vi "Untitled 2.vi"() -> ()   [LabVIEW 2020]
uses:
  HAL/Source/Communicator/Communicator.lvclass
  D:/git/HAL/Source/Interfaces/ICommunicate/ICommunicate.lvclass
  HAL/HAL-Devices/source/PCAN USB Dongle/PCAN Basic 4/Configure Strategies/Read-Write CAN Frame Strategy/PCAN Basic4 Read-Write CAN CC Frame Strategy.lvclass
  D:/git/HAL/Source/Interfaces/IConfigure/IConfigure.lvclass
  HAL/Source/Interfaces/IMessage/IMessage.lvclass
  source/SDO Manager/SDO Manager/SDO Manager.lvclass
  source/SDO Manager/SDO Transfer/SDO abort code.ctl
  source/SDO Manager/SDO Transfer/SDO Transfer.lvclass
  source/Typedefs/SDO Result.ctl
  source/CANopen.lvlib
panel:
  out "(hi.lo)":u32
  out "Data R":u8[](array[numeric]) format="%x"
  out "Data S":u8[](array[numeric]) format="%x"
  out "SDO Result":T1={"Success"=FALSE, "SDO abort code"={"Null"=TRUE, "Value"=84082688}, "Data"={"Null"=TRUE, "Data"=[]}} {"SDO abort code"."Value" items=["Toggle bit not allowed"=84082688, "SDO protocol timed out"=84148224, "Client/server command specifier not valid or unknown"=84148225, "Invalid block size (block mode only)"=84148226, "Invalid sequence number (block mode only)"=84148227, "CRC error (block mode only)"=84148228, "Out of memory"=84148229, "Attempt to read a write only object"=100728833, "Attempt to write a read only object"=100728834, "Object does not exist in the object dictionary"=100794368, "Object cannot be mapped to the PDO"=100925505, "The number and length of the objects to be mapped would exceed PDO length"=100925506, "General parameter incompatibility reason"=100925507, "General internal incompatibility in the device"=100925511, "Access failed due to an hardware error"=101056512, "Data type does not match, length of service parameter does not match"=101122064, "Data type does not match, length of service parameter too high"=101122066, "Data type does not match, length of service parameter too low"=101122067, "Sub-index does not exist"=101253137, "Invalid value for parameter (download only)"=101253168, "Value of parameter written too high (download only)"=101253169, "Value of parameter written too low (download only)"=101253170, "Maximum value is less than minimum value"=101253174, "Resource not available: SDO connection"=101318691, "General error"=134217728, "Data cannot be transferred or stored to the application"=134217760, "Data cannot be transferred or stored to the application because of local control"=134217761, "Data cannot be transferred or stored to the application because of the present device stable"=134217762, "Object dictionary dynamic generation fails or no object dictionary is present (e.g. object dictionary is generated from file and generation fails because of an file error)"=134217763, "No data available"=134217764]; "Data"."Data" format="%02x"}
  out "error out":errorcluster
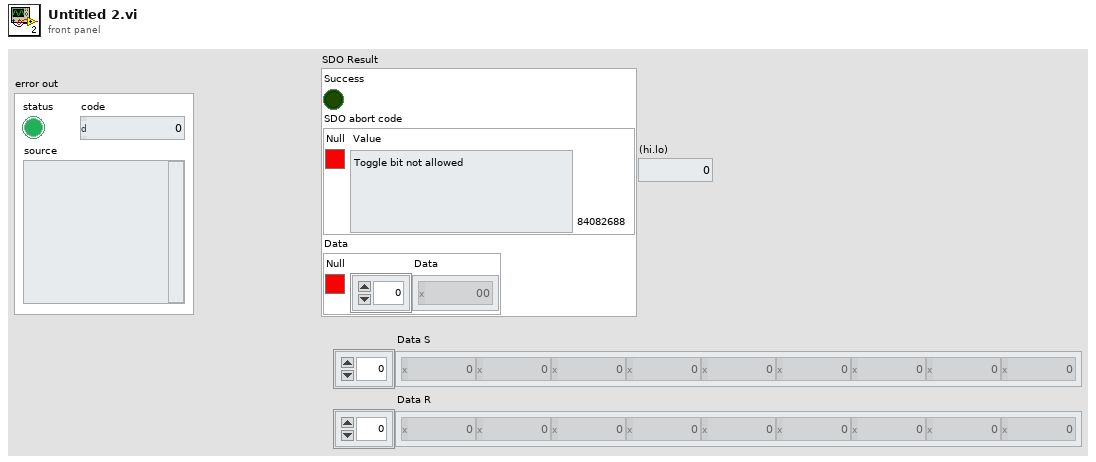
[diagram p1: front panel]
types:
  T1 = typedef "CANopen.lvlib/SDO Result.ctl" = cluster{"Success":bool, "SDO abort code":cluster{"Null":bool, "Value":T2}, "Data":cluster{"Null":bool, "Data":u8[]}}
  T2 = typedef "SDO Manager.lvlib/SDO Transfer.lvclass/SDO abort code.ctl" = u32
  T3 = cluster{"Node-ID":u8, "Multiplexer":cluster{"Index":u16, "Sub-Index":u8}, "Data":u8[]}
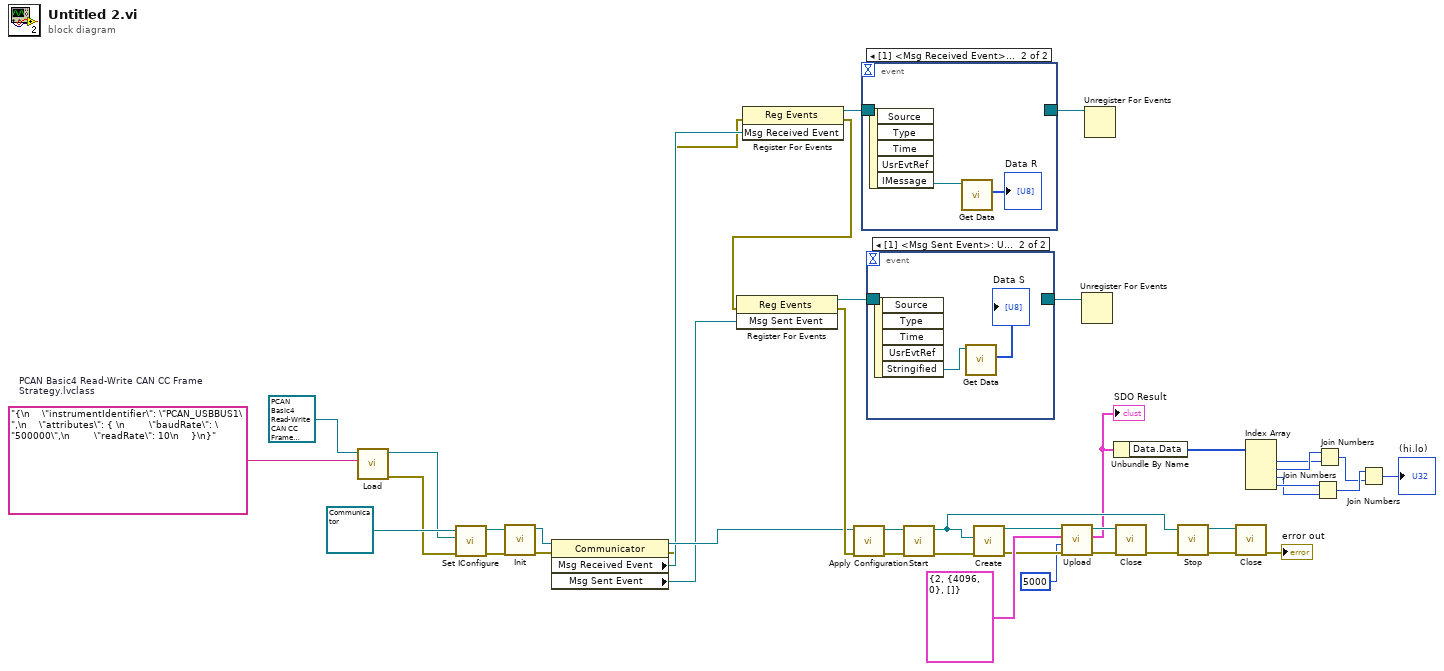
[diagram p0: block diagram]
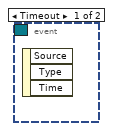
[diagram p2: hidden frame]
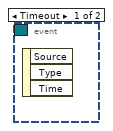
[diagram p3: hidden frame]
diagram:
  w42 = refnum<class "PCAN Basic4 Read-Write CAN CC Frame Strategy.lvclass"> refnum  # PCAN Basic4 Read-Write CAN CC Frame Strategy.lvclass
  n1 = call-dynamic "Load.vi"("Source"="{\n    \"instrumentIdentifier\": \"PCAN_USBBUS1\",\n    \"attributes\": { \n        \"baudRate\": \"500000\",\n        \"readRate\": 10\n    }\n}", "PCAN Basic Base Configure Strategy in"=w42) -> ("error out"=w21:errorcluster, "PCAN Basic Base Configure Strategy out"=w22:refnum<class "PCAN Basic4 Read-Write CAN CC Frame Strategy.lvclass">)  [unwired: 8 in]
  n2 = call-dynamic "Set IConfigure.vi"("Error In"=w21, "IConfigure"=w22, "Communicator in"=refnum<class "Communicator.lvclass"> refnum ("Communicator")) -> ("Error Out"=w35:errorcluster, "Communicator out"=w36:refnum<class "Communicator.lvclass">)  [unwired: 7 in]
  n3 = call-dynamic "Init.vi"("Error In"=w35, "Communicator in"=w36) -> ("Error Out"=w34:errorcluster, "Communicator out"=w20:refnum<class "Communicator.lvclass">)  [unwired: 8 in]
  n4 = property class="Communicator"(reference=w20, error in=w34) -> (reference out=w17:refnum<class "Communicator.lvclass">, error out=w11:errorcluster, "Msg Received Event"=w14:refnum<user-event>, "Msg Sent Event"=w16:refnum<user-event>)
  n5 = register-events(error in=w11, w14) -> (reference out=w15:refnum<event-registration>, error out=w10:errorcluster)  [unwired: 1 in]
  n6 = register-events(error in=w10, w16) -> (reference out=w19:refnum<event-registration>, error out=w18:errorcluster)  [unwired: 1 in]
  n7 = call-dynamic "Apply Configuration.vi"("Error In"=w18, "Communicator in"=w17) -> ("Error Out"=w41:errorcluster, "Communicator out"=w40:refnum<class "Communicator.lvclass">)  [unwired: 8 in]
  n8 = event shown="[1] <Msg Received Event>: User Event" {
    selector: w15 -> [_ _]
    dyn-events: [_ _] -> w12
    timeout: _ -> [_ _]
    event Timeout {
      n9 = event-data() -> ()  [unwired: 1 in, 3 out]
    }
    event User Event {
      n10 = event-data() -> ("IMessage"=w44:refnum<class "IMessage.lvclass">)  [unwired: 1 in, 4 out]
      n11 = call-dynamic "Get Data.vi"("IMessage in"=w44) -> ("Data"=→"Data R":u8[])  [unwired: 8 in, 2 out]
    }
  }
  n12 = event shown="[1] <Msg Sent Event>: User Event" {
    selector: w19 -> [_ _]
    dyn-events: [_ _] -> w13
    timeout: _ -> [_ _]
    event Timeout {
      n13 = event-data() -> ()  [unwired: 1 in, 3 out]
    }
    event User Event {
      n14 = event-data() -> ("Stringified"=w45:refnum<class "IMessage.lvclass">)  [unwired: 1 in, 4 out]
      n15 = call-dynamic "Get Data.vi"("IMessage in"=w45) -> ("Data"=→"Data S":u8[])  [unwired: 8 in, 2 out]
    }
  }
  n16 = call-dynamic "Start.vi"("Error In"=w41, "Communicator in"=w40) -> ("Error Out"=w39:errorcluster, "Communicator out"=w29:refnum<class "Communicator.lvclass">)  [unwired: 8 in]
  n17 = call "Create.vi"("Error In"=w39, "ICommunicate"=w29) -> ("Error Out"=w26:errorcluster, "SDO Manager"=w28:refnum<class "SDO Manager.lvclass">)  [unwired: 8 in]
  n18 = call "Upload.vi"("Error In"=w26, "Timeout"=5000, "Parameters"=T3 {"Node-ID"=2, "Multiplexer"={"Index"=4096, "Sub-Index"=0}, "Data"=[]}, "SDO Manager in"=w28) -> ("Error Out"=w25:errorcluster, "SDO Result"=w9:T1, "SDO Manager out"=w24:refnum<class "SDO Manager.lvclass">)  [unwired: 5 in]
  "SDO Result" <- w9
  n19 = Unregister For Events(event registration refnum=w13) -> ()  [unwired: 1 in, 1 out]
  n20 = Unregister For Events(event registration refnum=w12) -> ()  [unwired: 1 in, 1 out]
  n21 = Unbundle By Name(w9) -> ("Data.Data"=w8:u8[])
  n22 = call "Close.vi"("Error In"=w25, "SDO Manager"=w24) -> ("Error Out"=w33:errorcluster)  [unwired: 8 in, 1 out]
  n23 = call-dynamic "Stop.vi"("Error In"=w33, "Communicator in"=w29) -> ("Error Out"=w38:errorcluster, "Communicator out"=w30:refnum<class "Communicator.lvclass">)  [unwired: 8 in]
  n24 = call-dynamic "Close.vi"("Error In"=w38, "Communicator in"=w30) -> ("Error Out"=→"error out":errorcluster)  [unwired: 8 in, 1 out]
  n25 = Index Array(array=w8) -> (element #1=w4:u8, element #2=w5:u8, element #3=w6:u8, element #4=w7:u8)  [unwired: 4 in]
  n26 = Join Numbers(hi=w7, lo=w6) -> ((hi.lo)=w3:u16)
  n27 = Join Numbers(hi=w5, lo=w4) -> ((hi.lo)=w2:u16)
  n28 = Join Numbers(hi=w3, lo=w2) -> ((hi.lo)=→"(hi.lo)":u32)
